vi "_CompareConnectorInfo.vi"(8 "error in (no error)":errorcluster, 10 "Cluster":T1, 11 "Cluster":T1) -> (0 "error out":errorcluster, 1 "Matched":bool, 2 "Cluster":T1, 3 "Cluster":T1)   [LabVIEW 2019, in "LabVIEW-ProviderShell.lvlib" / "LvProviderShellHelper.lvclass"]
uses:
  LvProviderShellHelper.lvclass
  def-ConnectorInfo.ctl
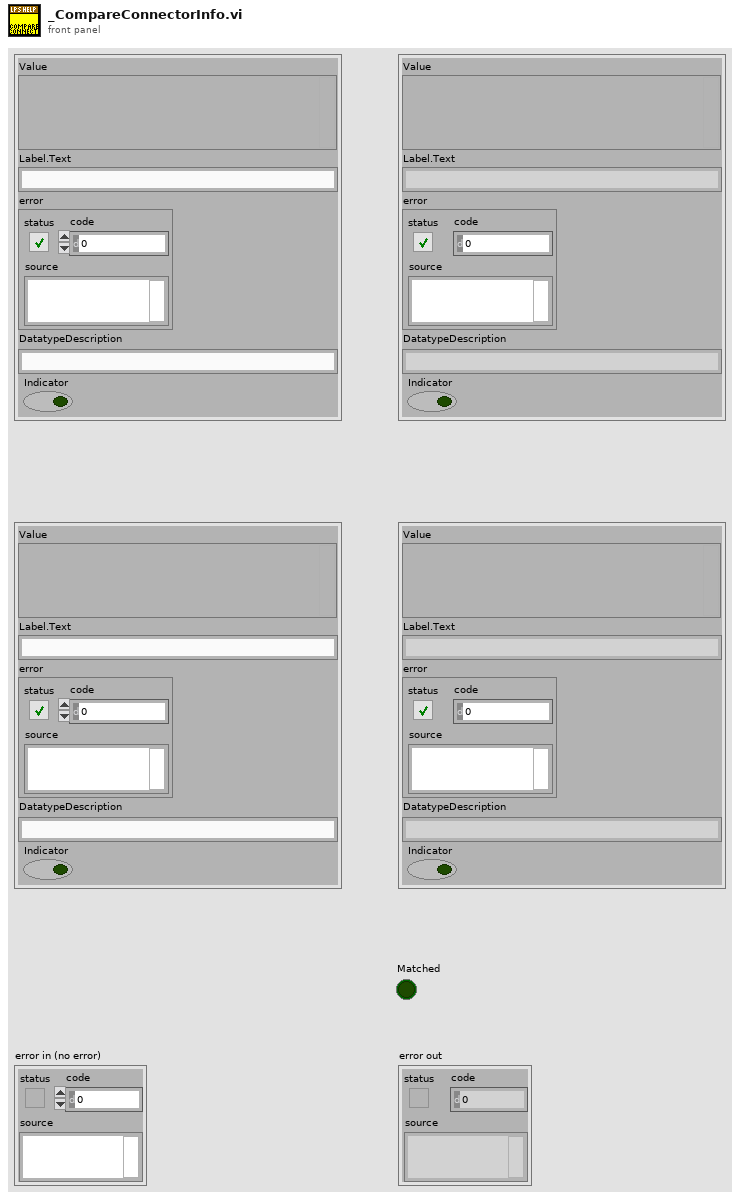
[diagram p1: front panel]
types:
  T1 = typedef "LabVIEW-ProviderShell.lvlib/LvProviderShellHelper.lvclass/def-ConnectorInfo.ctl" = cluster{"Value":variant, "Label.Text":string, "error":errorcluster, "DatatypeDescription":string, "Indicator":bool}
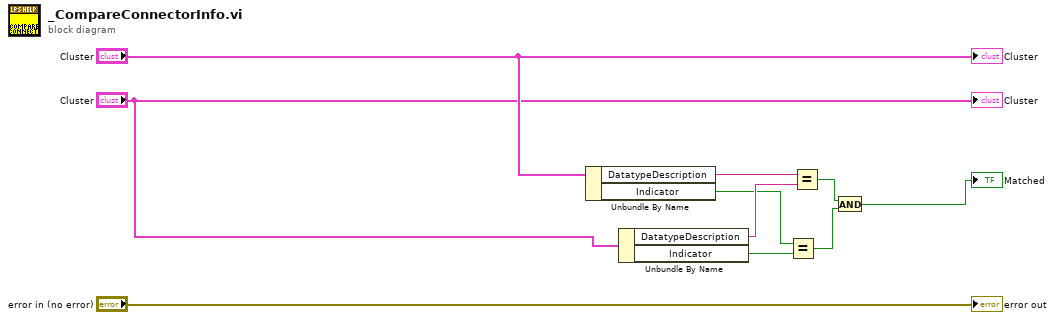
[diagram p0: block diagram]
diagram:
  n1 = Unbundle By Name("Cluster") -> ("DatatypeDescription"=w6:string, "Indicator"=w4:bool)
  n2 = Unbundle By Name("Cluster") -> ("DatatypeDescription"=w5:string, "Indicator"=w3:bool)
  n3 = Equal?(x=w4, y=w3) -> (x = y?=w2:bool)
  n4 = Equal?(x=w6, y=w5) -> (x = y?=w1:bool)
  n5 = And(x=w1, y=w2) -> (x .and. y?=→"Matched":bool)
  "error out" <- "error in (no error)"
  "Cluster" <- "Cluster"
  "Cluster" <- "Cluster"
